vi "Read Reset.vi"(8 "error in (no error)":errorcluster, 11 "FPGA VI Reference in":T1) -> (0 "error out":errorcluster, 2 "Reset":bool, 3 "FPGA VI Reference out":T1)   [LabVIEW 2009]
uses:
  TypeDefs/Sensor TypeDefs/FPGA Main ref.ctl
  <vilib>/rvi/interface/nirviReadWriteControl/nirviReadWriteControl.xnode
  FPGA Bitfiles/Q_IGVC_2010.lvproj_FPGA Target_FPGA_MAIN.vi.lvbitx
  <vilib>/Utility/error.llb/Error Cluster From Error Code.vi
  <vilib>/rvi/errors/niLvFpgaAdjustHostInterfaceError.vi
  <vilib>/rvi/interface/common/niFpgaNodeNameForErrorReporting.ctl
  <vilib>/rvi/errors/niLvFpgaWhatHappensToTopLevelVI.ctl
  NiRioSrv.dll
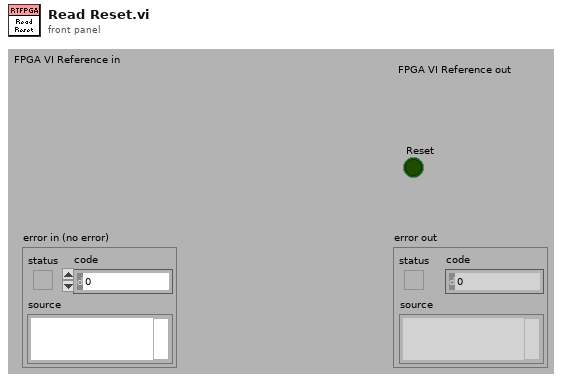
[diagram p1: front panel]
types:
  T1 = typedef "FPGA Main ref.ctl" = refnum<k20>
  T2 = typedef "niFpgaNodeNameForErrorReporting.ctl" = enum16{"Open FPGA VI Reference", "Read/Write Control", "Invoke Method: Abort", "Invoke Method: Acknowledge IRQ", "Invoke Method: Download", "Invoke Method: FIFO.Configure", "Invoke Method: FIFO.Read", "Invoke Method: FIFO.Start", "Invoke Method: FIFO.Stop", "Invoke Method: FIFO.Write", "Invoke Method: Reset", "Invoke Method: Run", "Invoke Method: Wait on IRQ", "Close FPGA VI Reference"}
  T3 = typedef "niLvFpgaWhatHappensToTopLevelVI.ctl" = enum16{"top level VI scripted behind XNode", "top level VI inlined behind XNode"}
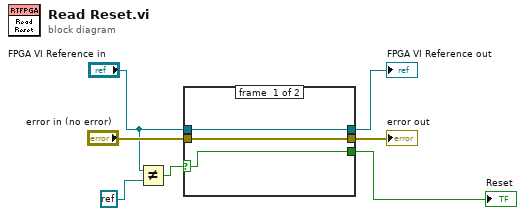
[diagram p0: block diagram]
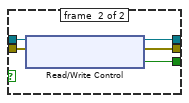
[diagram p2: hidden frame]
diagram:
  n1 = Not Equal?(x="FPGA VI Reference in", y=refnum<k0> refnum) -> (x != y?=w3:bool)
  n2 = case shown="False" w3 {
    selector: w3 -> [w8 _]
    tunnel: [w8 w15] -> w7
    tunnel: [w10 w14] -> w6
    tunnel: [w9 w13] -> w5
    tunnel: "error in (no error)" -> [w9 w12]
    tunnel: "FPGA VI Reference in" -> [w10 w11]
    frame #0 {
    }
    frame #1 {
      n3 = xnode "Read/Write Control"("FPGA VI Reference In"=w11, "error in"=w12) -> ("FPGA VI Reference Out"=w14:T1, "error out"=w13:errorcluster, "Debounced BTTN1"=w15:bool)
    }
  }
  "FPGA VI Reference out" <- w6
  "error out" <- w5
  "Reset" <- w7
